vi "Get Window Name.vi"(8 "error in (no error)":errorcluster, 11 "window refnum in (NaWR)":T1) -> (0 "error out":errorcluster, 2 "window name":string, 3 "window refnum out":T1)   [LabVIEW 2020, in "MacroAssert.lvlib" / "WINUTIL.lvlib"]
doc: "This VI will use window refnum in to get the name of a window. The name of a window is simply the text appearing in the title bar of the window. If the title bar of the window is not shown, the name of the window will be a NULL string."
uses:
  WINUTIL.lvlib
  Window Refnum.ctl
  user32.dll
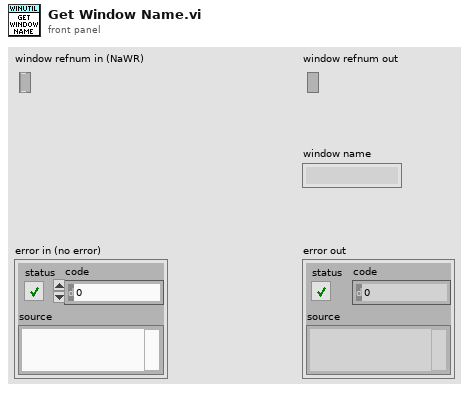
[diagram p1: front panel]
types:
  T1 = typedef "MacroAssert.lvlib/WINUTIL.lvlib/Window Refnum.ctl" = refnum<k1>
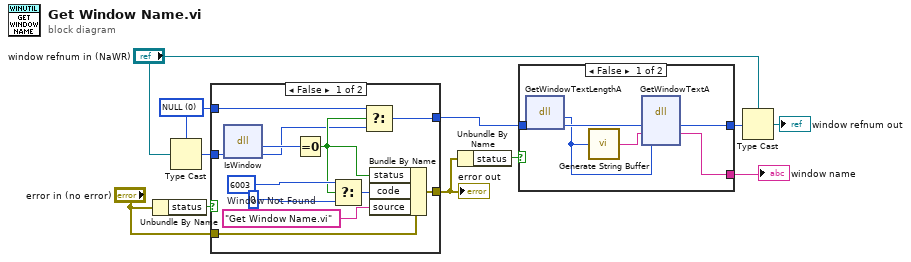
[diagram p0: block diagram]
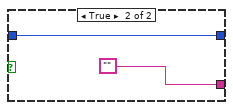
[diagram p2: hidden frame]
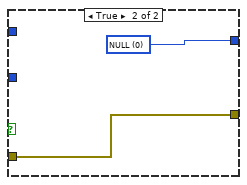
[diagram p3: hidden frame]
diagram:
  w1 = u32 0 items=["NULL"]
  n1 = Unbundle By Name("error in (no error)") -> ("status"=w11:bool)
  n2 = Type Cast(type=w1, x="window refnum in (NaWR)") -> (*(type *) &x=w5:u32)
  n3 = case shown="False" w11 {
    tunnel: "error in (no error)" -> [w14 w24]
    tunnel: w5 -> [w23 _]
    tunnel: [w15 w25] -> w8
    tunnel: [w13 w24] -> w7
    tunnel: w1 -> [w12 _]
    frame False {
      w20 = 6003  # Window Not Found
      n4 = dll-call lib="user32.dll" fn="IsWindow"("hWnd"=w23) -> ("IsWindow?"=w22:i32, "hWnd"=w16:u32)  [unwired: 3 in, 2 out]
      n5 = Equal To 0?(x=w22) -> (x = 0?=w17:bool)
      n6 = Select(t=w20, s=w17, f=0) -> (s? t:f=w19:i32)
      n7 = Select(t=w12, s=w17, f=w16) -> (s? t:f=w15:u32)
      n8 = Bundle By Name(cluster=w14, "status"=w17, "code"=w19, "source"="Get Window Name.vi") -> (w13:errorcluster)
    }
    frame True {
      w25 = u16 0 items=["NULL"]
    }
  }
  "error out" <- w7
  n9 = Unbundle By Name(w7) -> ("status"=w9:bool)
  n10 = case shown="False" w9 {
    tunnel: w8 -> [w29 w32]
    tunnel: [w31 w32] -> w3
    tunnel: [w30 ""] -> w6
    frame False {
      n11 = dll-call lib="user32.dll" fn="GetWindowTextLengthA" label="GetWindowTextLength"("hWnd"=w29) -> ("length"=w27:i32, "hWnd"=w28:u32)  [unwired: 3 in, 2 out]
      n12 = call "Generate String Buffer.vi"("buffer size"=w27) -> ("string buffer"=w26:string)
      n13 = dll-call lib="user32.dll" fn="GetWindowTextA" label="GetWindowText"("hWnd"=w28, "NameBuffer"=w26, "MaxCharsToCopy"=w27) -> ("hWnd"=w31:u32, "NameBuffer"=w30:string)  [unwired: 4 in, 3 out]
    }
    frame True {
    }
  }
  "window name" <- w6
  n14 = Type Cast(type="window refnum in (NaWR)", x=w3) -> (*(type *) &x=→"window refnum out":T1)
